vi "ChipKit Photocell.vi"() -> ()   [LabVIEW 2011, in "LabVIEW Interface for ChipKit.lvlib"]
doc: "An example that reads a user selectable analog input pin on the ChipKit."
uses:
  vi.lib/LabVIEW Interface for ChipKit/LabVIEW Interface for ChipKit.lvlib
  vi.lib/LabVIEW Interface for ChipKit/Private/Type Defs/Chipkit Resource.ctl
  vi.lib/LabVIEW Interface for ChipKit/Private/Type Defs/Board Type.ctl
  vi.lib/LabVIEW Interface for ChipKit/Private/Type Defs/Connection Type.ctl
  vi.lib/LabVIEW Interface for ChipKit/Private/Type Defs/Analog Pin.ctl
panel:
  in  "Photocell Pin":T1=enum."AI_1"
  out "Waveform Chart":dbl(graph)=57.8312
  in  "Stop Button":bool
  in  "ChipKit Configuration":T2={"COM Port"="COM3", "Board Type"=enum."ChipKit uC32", "Connection Type"=enum."USB / Serial", "Baud Rate (115200)"=115200, "Bytes Per Packet (15)"=15}
  # "Photocell Read Example\n\nThis example demonstrates how to measure light intensity using a photocell.  The light intensity output ranges from 0 in complete \ndarkness to 100 in direct light.\n\nInstructions\n1. Select the COM Port associated with the ChipKit.\n2. Select the Board Type.\n3. Select the Photocell Pin to read from.\n4. Click the Run Arrow.\n5. Adjust the amount of light shining on the photocell."
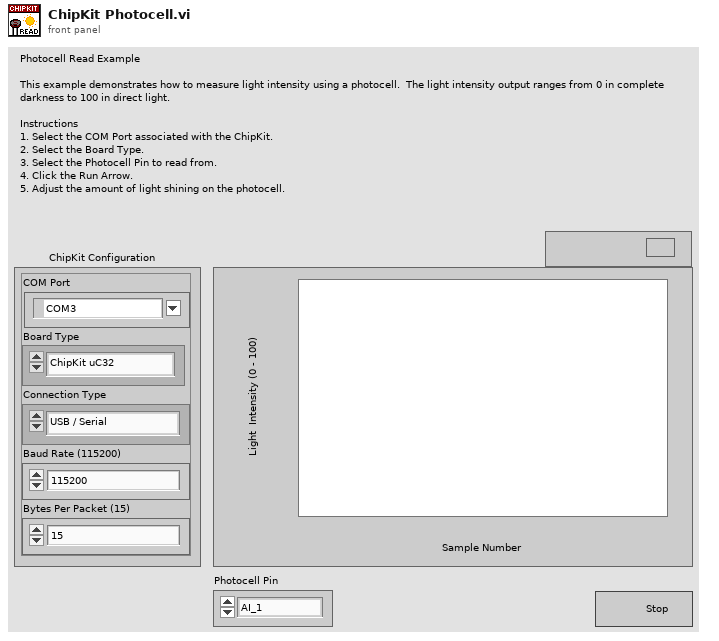
[diagram p1: front panel]
types:
  T1 = typedef "LabVIEW Interface for ChipKit.lvlib/Analog Pin.ctl" = enum16{"AI_0", "AI_1", "AI_2", "AI_3", "AI_4", "AI_5", "AI_6", "AI_7", "AI_8", "AI_9", "AI_10", "AI_11", "AI_12", "AI_13", "AI_14", "AI_15"}
  T2 = typedef "LabVIEW Interface for ChipKit.lvlib/Chipkit Resource.ctl" = cluster{"COM Port":refnum<visa-resource-name>, "Board Type":T3, "Connection Type":T4, "Baud Rate (115200)":u32, "Bytes Per Packet (15)":u32}
  T3 = typedef "LabVIEW Interface for ChipKit.lvlib/Board Type.ctl" = enum16{"ChipKit uC32", "ChipKit Uno32", "ChipKit Max32"}
  T4 = typedef "LabVIEW Interface for ChipKit.lvlib/Connection Type.ctl" = enum8{"USB / Serial", "XBEE", "BlueSmirf (Bluetooth)"}
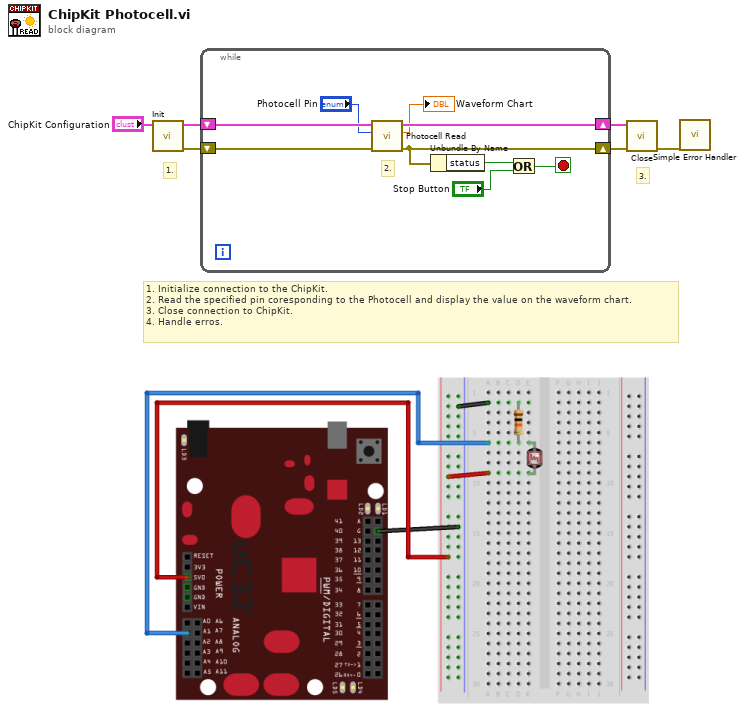
[diagram p0: block diagram]
diagram:
  # "1. Initialize connection to the ChipKit.\n2. Read the specified pin coresponding to the Photocell and display the value on the waveform chart.\n3. Close connection to ChipKit.\n4. Handle erros."
  # "3."
  # "1."
  n1 = call "Init.vi"("ChipKit Configuration"="ChipKit Configuration") -> ("Error Out"=w3:errorcluster, "ChipKit Configuration"=w6:T2)  [unwired: 9 in]
  n2 = while {
    shift-right: [w15] -> w5
    shift-left: w6 -> [w11]
    shift-right: [w14] -> w4
    shift-left: w3 -> [w10]
    stop <- w13 stop-if-true
    # "2."
    n3 = call "Photocell Read.vi"("Error In"=w10, "Photocell Pin (0)"="Photocell Pin", "ChipKit Resource"=w11) -> ("Error Out"=w14:errorcluster, "Light Intensity (0 - 100)"=→"Waveform Chart":dbl, "ChipKit Resource"=w15:T2)  [unwired: 6 in]
    n4 = Unbundle By Name(w14) -> ("status"=w12:bool)
    n5 = Or(x=w12, y="Stop Button") -> (x .or. y?=w13:bool)
  }
  n6 = call "Close.vi"("Error In"=w4, "ChipKit Configuration"=w5) -> ("Error Out"=w2:errorcluster)  [unwired: 9 in]
  n7 = call <vilib>:"Simple Error Handler.vi"("error in (no error)"=w2) -> ()  [unwired: 4 in, 5 out]
